vi "global.vi"() -> ()   [LabVIEW 2017]
panel:
  out "motion_command":bool
  in  "Torque_R":dbl
  in  "Speed_R":dbl
  out "RC received":bool
  in  "CTL_mode":u8
  in  "Torque_L":dbl
  in  "Speed_L":dbl
  in  "RC Control":bool
  out "Speed/Torque":bool
  in  "Stop":bool
  out "error":bool
  in  "rc_ch2":dbl
  in  "rc_ch1":dbl
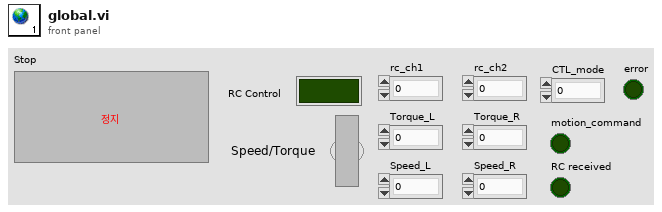
[diagram p1: front panel]
diagram:
